vi "GooglePlatform OAuth Test.vi"() -> ()   [LabVIEW 2017]
uses:
  Oauth2/Oauth2.lvclass/Oauth2.ctl
  Oauth2.Google/Oauth2.Google.lvclass
  D:/GitHub/Oauth2/source/Oauth2/Oauth2.lvclass
  Oauth2/Read RefreshToken.vi
  Oauth2/Read ExpiresIn.vi
  Oauth2/Read Redirect URI.vi
  Oauth2/Read scopes.vi
  <vilib>/dlg_ctls.llb/Space Constant.vi
  OAuthToken/Retrieve Element.vi
  Oauth2/Oauth2.lvclass
  <vilib>/LabVIEW Open Source Project/OpenURI/uri/URI.lvclass
  <vilib>/httpClient/LabVIEWHTTPClient.lvlib
  JWT/JSONWebToken.lvclass
panel:
  out "Valid JWT?":bool
  in  "relative API URI":string="userinfo/v2/me"
  out "REST API Error":errorcluster
  in  "Query API Version":bool
  in  "Refresh":bool
  in  "Authorize":bool
  out "API Response":string
  out "HTTP Response Headers":string
  out "Redirect URI":string
  out "scopes":string[](array[string])
  out "Expires In":u32
  out "Refresh Token":string
  in  "Google Client Secret":string="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"
  in  "Google Client ID":string="84373447473-896ics1sdlo85ltm2vc5tflvgn2h9se5.apps.googleusercontent.com"
  out "Google Access Token":string
  out "Oauth Error":errorcluster
  # "Google Cloud Application API Access Example"
  # "G Open Source Project for LabVIEW\nhttps://github.com/LabVIEW-Open-Source/Oauth2"
  # "1- Get a Client ID and Client Secret from the application's admin. \n\n          * To access your own server, log into your site, create an application and set the access scope.\n             you want. \n          * This Oauth2.0 API uses the following redirect URL: http://localhost:58888/Oauth2/Redirect\n          * Record the client ID and client secret and fill in the fields below."
  # "2- Get an Access Token. You will be redirected your Google's Authorization Server URI\n              * Use the \"Get Access Token\" button on the top right of this page.\n\n3- Once you have authenticated yourself, you will receive an access token.\n              * Use the \"Refresh Token\" button to request a fresh token\n                       OR\n              * Use the Access Token to query the Google API (example is to retrieve the User Info)\n\n4- Visit \"https://developers.google.com/oauthplayground/\" if you'd like to run Oauth2 tests."
  # "0: Never expired"
  # "https://www.googleapis.com/"
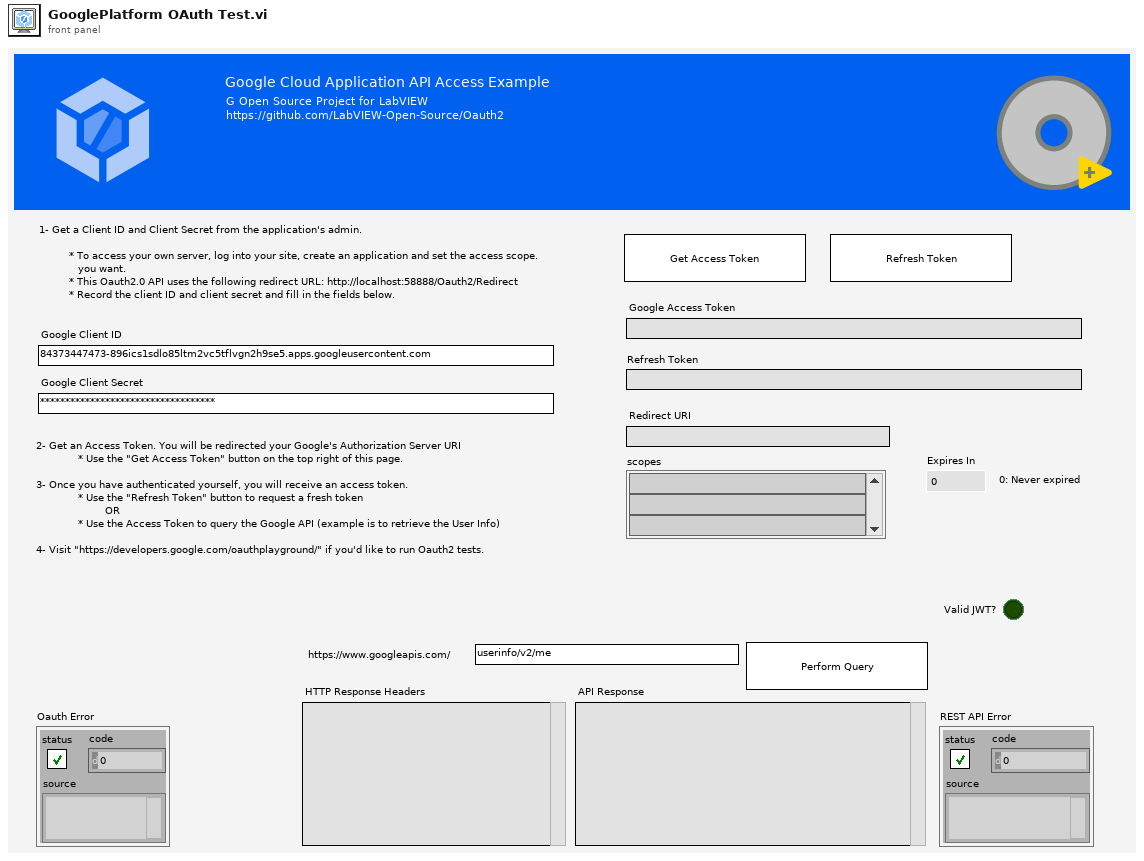
[diagram p1: front panel]
types:
  T1 = enum8{"Enabled", "Disabled", "Disabled and Grayed Out"}
  T2 = typedef "LabVIEWHTTPClient.lvlib/ClientHandle.ctl" = refnum<k1>
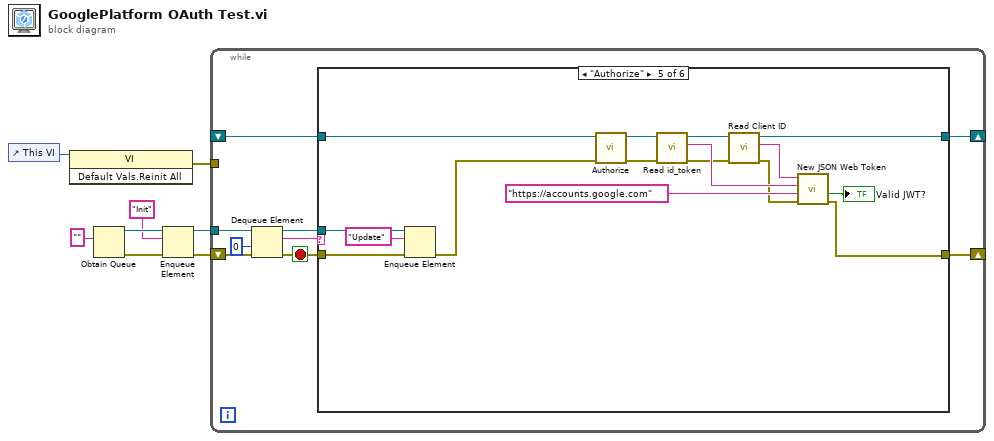
[diagram p0: block diagram]
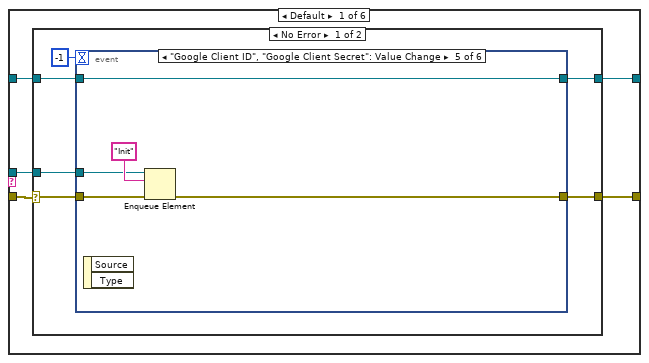
[diagram p2: hidden frame]
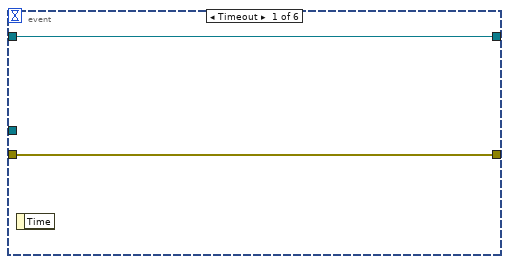
[diagram p3: hidden frame]
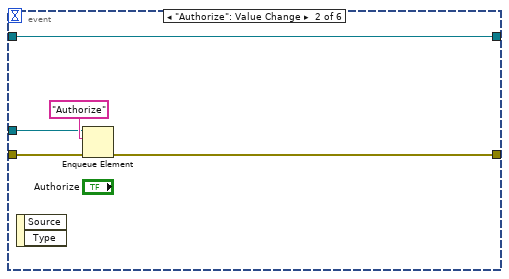
[diagram p4: hidden frame]
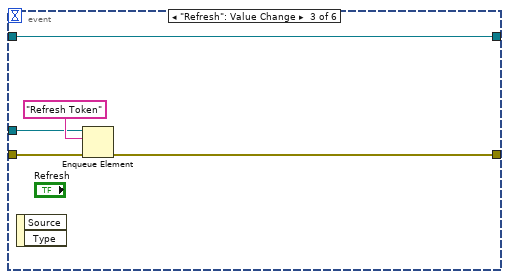
[diagram p5: hidden frame]
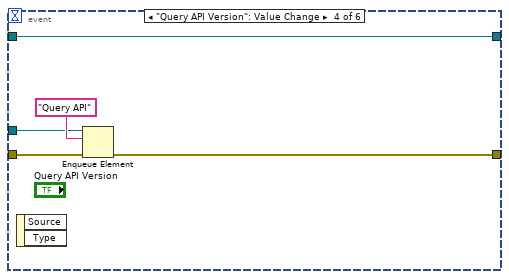
[diagram p6: hidden frame]
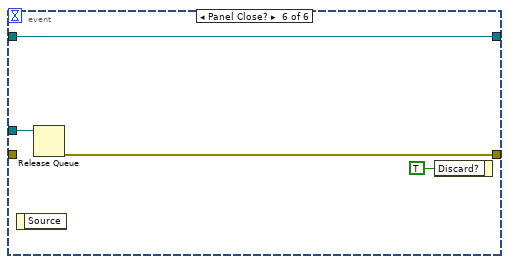
[diagram p7: hidden frame]
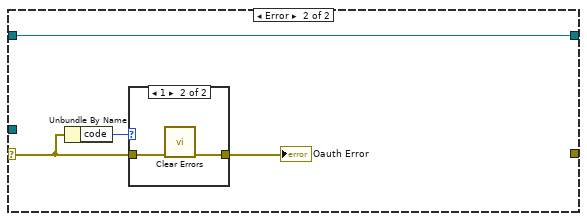
[diagram p8: hidden frame]
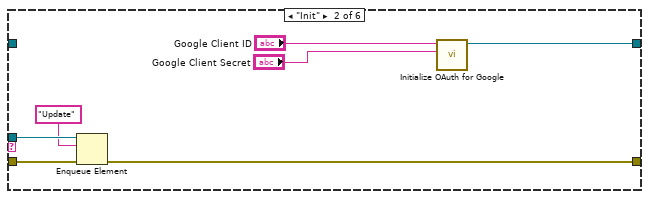
[diagram p10: hidden frame]
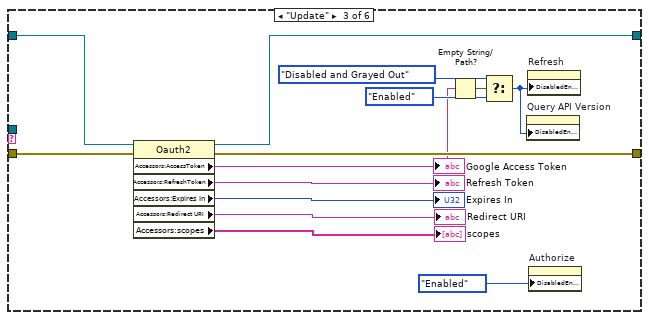
[diagram p11: hidden frame]
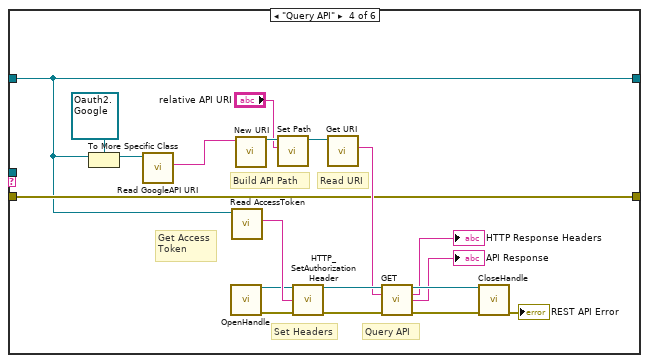
[diagram p12: hidden frame]
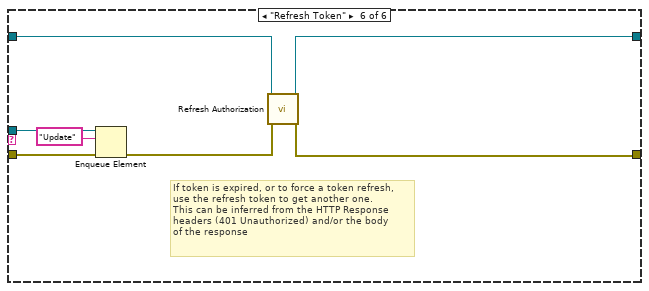
[diagram p13: hidden frame]
diagram:
  n1 = control-ref of="This VI"() -> (w1:refnum<vi>)
  n2 = invoke class="VI" method="Default Vals.Reinit All"(reference=w1) -> (error out=w2:errorcluster)  [unwired: 2 in, 2 out]
  n3 = Obtain Queue(element data type="") -> (queue out=w5:refnum<queue>, error out=w7:errorcluster)  [unwired: 4 in, 1 out]
  n4 = Enqueue Element(queue=w5, element="Init", error in (no error)=w7) -> (queue out=w4:refnum<queue>, error out=w6:errorcluster)  [unwired: 1 in, 1 out]
  n5 = while {
    tunnel: w4 -> [w17]
    shift-right: [w12] -> _
    shift-left: _ -> [w11]
    shift-right: [w9] -> _
    shift-left: w6 -> [w13]
    tunnel: w2 -> [_]
    stop <- w10 stop-if-true
    n6 = Dequeue Element(queue=w17, timeout in ms (-1)=0, error in (no error)=w13) -> (queue out=w14:refnum<queue>, element=w15:string, error out=w10:errorcluster)  [unwired: 1 out]
    n7 = case shown="\"Authorize\"" w15 {
      tunnel: w14 -> [w22 w68 _ _ w116 w123]
      tunnel: [w21 w62 w70 w84 w105 w118] -> w12
      tunnel: w11 -> [w20 _ w69 w84 w113 w119]
      tunnel: w10 -> [w19 w65 w79 w90 w115 w122]
      tunnel: [w18 w66 w78 w90 w107 w120] -> w9
      frame Default {
        n8 = case shown="No Error" w19 {
          selector: w19 -> [w23 w57]
          tunnel: w22 -> [w27 _]
          tunnel: [w26 w58] -> w21
          tunnel: w20 -> [w25 w58]
          tunnel: [w24 _] -> w18
          frame No Error {
            n9 = event shown="[4] \"Google Client ID\", \"Google Client Secret\": Value Change" {
              selector: _ -> [_ _ _ _ _ _]
              dyn-events: _ -> [_ _ _ _ _ _]
              timeout: -1 -> [_ _ _ _ _ _]
              tunnel: w27 -> [_ w34 w39 w44 w49 w54]
              tunnel: [w30 w32 w37 w42 w47 w52] -> w26
              tunnel: w25 -> [w30 w32 w37 w42 w47 w52]
              tunnel: [w29 w31 w36 w41 w46 w51] -> w24
              tunnel: w23 -> [w29 w33 w38 w43 w48 _]
              event Timeout {
                n10 = event-data() -> ()  [unwired: 1 in, 1 out]
              }
              event "Authorize": Value Change {
                n11 = event-data() -> ()  [unwired: 1 in, 2 out]
                n12 = Enqueue Element(queue=w34, element="Authorize", error in (no error)=w33) -> (error out=w31:errorcluster)  [unwired: 1 in, 2 out]
              }
              event "Refresh": Value Change {
                n13 = event-data() -> ()  [unwired: 1 in, 2 out]
                n14 = Enqueue Element(queue=w39, element="Refresh Token", error in (no error)=w38) -> (error out=w36:errorcluster)  [unwired: 1 in, 2 out]
              }
              event "Query API Version": Value Change {
                n15 = event-data() -> ()  [unwired: 1 in, 2 out]
                n16 = Enqueue Element(queue=w44, element="Query API", error in (no error)=w43) -> (error out=w41:errorcluster)  [unwired: 1 in, 2 out]
              }
              event "Google Client ID", "Google Client Secret": Value Change {
                n17 = event-data() -> ()  [unwired: 1 in, 2 out]
                n18 = Enqueue Element(queue=w49, element="Init", error in (no error)=w48) -> (error out=w46:errorcluster)  [unwired: 1 in, 2 out]
              }
              event Panel Close? {
                n19 = event-data() -> ()  [unwired: 1 in, 1 out]
                n20 = Release Queue(queue=w54) -> (error out=w51:errorcluster)  [unwired: 2 in, 2 out]
                n21 = event-data("Discard?"=TRUE) -> ()  [unwired: 1 in, 1 out]
              }
            }
          }
          frame Error {
            n22 = Unbundle By Name(w57) -> ("code"=w55:i32)
            n23 = case shown="1" w55 {
              tunnel: w57 -> [w59 w61]
              tunnel: [w59 w60] -> w56
              frame Default {
              }
              frame 1 {
                n24 = call <vilib>:"Clear Errors.vi"("error in (no error)"=w61) -> ("error out"=w60:errorcluster)  [unwired: 5 in, 1 out]
              }
            }
            "Oauth Error" <- w56
          }
        }
      }
      frame "Init" {
        n25 = Enqueue Element(queue=w68, element="Update", error in (no error)=w65) -> (error out=w66:errorcluster)  [unwired: 1 in, 2 out]
        n26 = call "Initialize OAuth for Google.vi"("Client Secret"="Google Client Secret", "Client ID"="Google Client ID") -> ("Oauth2.Google"=w62:refnum<class "Oauth2.Google.lvclass">)  [unwired: 8 in, 1 out]
      }
      frame "Update" {
        n27 = property class="Oauth2"(reference=w69, error in=w79) -> (reference out=w70:refnum<class "Oauth2.lvclass">, error out=w78:errorcluster, "Accessors:AccessToken"=w77:string, "Accessors:RefreshToken"=→"Refresh Token":string, "Accessors:Expires In"=→"Expires In":u32, "Accessors:Redirect URI"=→"Redirect URI":string, "Accessors:scopes"=→"scopes":string[])
        "Google Access Token" <- w77
        n28 = Empty String/Path?(string/path=w77) -> (empty?=w82:bool)
        n29 = Select(t=T1."Disabled and Grayed Out" ("Disabled"), s=w82, f=T1."Enabled" ("Disabled")) -> (s? t:f=w72:T1)
        n30 = property on="Query API Version" class="Bool"("DisabledEnum"=w72) -> ()  [unwired: 2 in, 2 out]
        n31 = property on="Refresh" class="Bool"("DisabledEnum"=w72) -> ()  [unwired: 2 in, 2 out]
        n32 = property on="Authorize" class="Bool"("DisabledEnum"=T1."Enabled" ("Disabled")) -> ()  [unwired: 2 in, 2 out]
      }
      frame "Query API" {
        # "Query API"
        # "Set Headers"
        # "Get Access\nToken"
        # "Read URI"
        # "Build API Path"
        n33 = To More Specific Class(target class=refnum<class "Oauth2.Google.lvclass"> refnum ("Oauth2.Google"), reference=w84) -> (specific class reference=w83:refnum<class "Oauth2.Google.lvclass">)  [unwired: 1 in, 1 out]
        n34 = call-dynamic "Read GoogleAPI URI.vi"("Oauth2.Google in"=w83) -> ("Token Server URI"=w86:string)  [unwired: 8 in, 2 out]
        n35 = call <vilib>:"OpenHandle.vi"() -> ("client handle out"=w100:T2, "error out"=w95:errorcluster)  [unwired: 14 in]
        n36 = call "Read AccessToken.vi"("Oauth2 in"=w84) -> ("Access Token"=w101:string)  [unwired: 8 in, 2 out]
        n37 = call <vilib>:"New URI.vi"("URI"=w86) -> ("URI"=w98:refnum<class "URI.lvclass">)  [unwired: 9 in, 1 out]
        n38 = call <vilib>:"Set Path.vi"("path"="relative API URI", "URI in"=w98) -> ("URI out"=w99:refnum<class "URI.lvclass">)  [unwired: 8 in, 1 out]
        n39 = call "HTTP_SetAuthorizationHeader.vi"("Client Handle"=w100, "Access Token"=w101, "error in (no error)"=w95) -> ("client handle dup"=w97:T2, "error out"=w94:errorcluster)  [unwired: 11 in]
        n40 = call <vilib>:"Get URI.vi"("URI in"=w99) -> ("URI String"=w96:string)  [unwired: 8 in, 2 out]
        n41 = call <vilib>:"GET.vi"("client handle"=w97, "url"=w96, "error in (no error)"=w94) -> ("client handle out"=w93:T2, "headers"=→"HTTP Response Headers":string, "body"=→"API Response":string, "error out"=w92:errorcluster)  [unwired: 9 in]
        n42 = call <vilib>:"CloseHandle.vi"("client handle"=w93, "error in (no error)"=w92) -> ("error out"=→"REST API Error":errorcluster)  [unwired: 13 in]
      }
      frame "Authorize" {
        n43 = Enqueue Element(queue=w116, element="Update", error in (no error)=w115) -> (error out=w114:errorcluster)  [unwired: 1 in, 2 out]
        n44 = call "Authorize.vi"("error in (no error)"=w114, "Oauth2 in"=w113) -> ("error out"=w108:errorcluster, "Oauth2 out"=w112:refnum<class "Oauth2.lvclass">)  [unwired: 7 in, 1 out]
        n45 = call "Read id_token.vi"("error in (no error)"=w108, "Oauth2 in"=w112) -> ("error out"=w104:errorcluster, "id_token"=w111:string, "Oauth2 out"=w106:refnum<class "Oauth2.lvclass">)  [unwired: 7 in]
        n46 = call "Read Client ID.vi"("error in (no error)"=w104, "Oauth2 in"=w106) -> ("error out"=w103:errorcluster, "Client ID"=w102:string, "Oauth2 out"=w105:refnum<class "Oauth2.lvclass">)  [unwired: 7 in]
        n47 = call "New JSON Web Token.vi"("error in (no error)"=w103, "Issuer URI path (component)"="https://accounts.google.com", "Base64url JWT string"=w111, "Client ID"=w102) -> ("error out"=w107:errorcluster, "Valid JWT?"=→"Valid JWT?":bool)  [unwired: 2 in, 4 out]
      }
      frame "Refresh Token" {
        # "If token is expired, or to force a token refresh, \nuse the refresh token to get another one.\nThis can be inferred from the HTTP Response\nheaders (401 Unauthorized) and/or the body\nof the response"
        n48 = Enqueue Element(queue=w123, element="Update", error in (no error)=w122) -> (error out=w121:errorcluster)  [unwired: 1 in, 2 out]
        n49 = call "Refresh Authorization.vi"("error in (no error)"=w121, "Oauth2 in"=w119) -> ("error out"=w120:errorcluster, "Oauth2 out"=w118:refnum<class "Oauth2.lvclass">)  [unwired: 7 in, 1 out]
      }
    }
  }
